vi "CSM - Read Log Filter Rules from INI Strings.vi"   [LabVIEW 2017, in "INI-Static-Variable-Support.lvlib"]
doc: "Reads log filter rules from the configuration. This configuration is primarily used with the following VIs:\n\n- `CSM - Set Log Filter Rules.vi`\n- `addons\\Logger\\CSM - Start File Logger.vi`"
uses:
  INI-Static-Variable-Support.lvlib
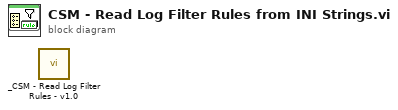
[diagram p0: block diagram]
diagram:
  n1 = call "_CSM - Read Log Filter Rules - v1.0.vi"() -> ()  [unwired: 8 in, 2 out]
